vi "G#Object_Create.vi"(0 "reference in":refnum<class "G#BaseAggregator.lvclass">, 3 "control values":variant[](array[variant]), 5 "error in (no error)":errorcluster) -> (14 "reference out":refnum<class "G#BaseAggregator.lvclass">, 19 "error out":errorcluster)   [LabVIEW 2017, in "G#BaseAggregator.lvclass"]
uses:
  G#BaseAggregator.lvclass
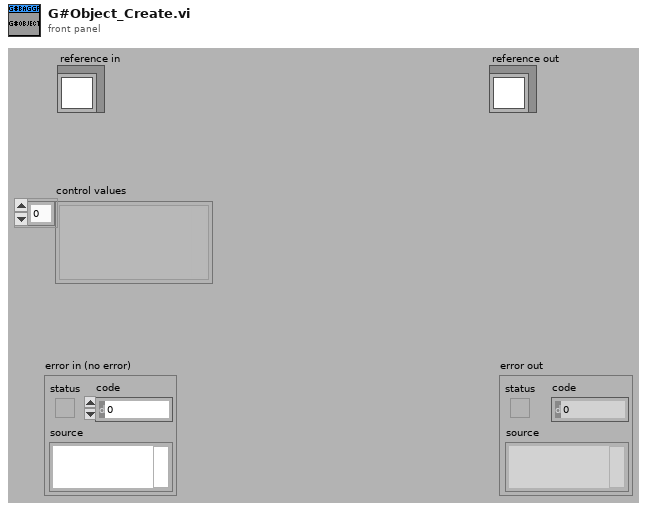
[diagram p1: front panel]
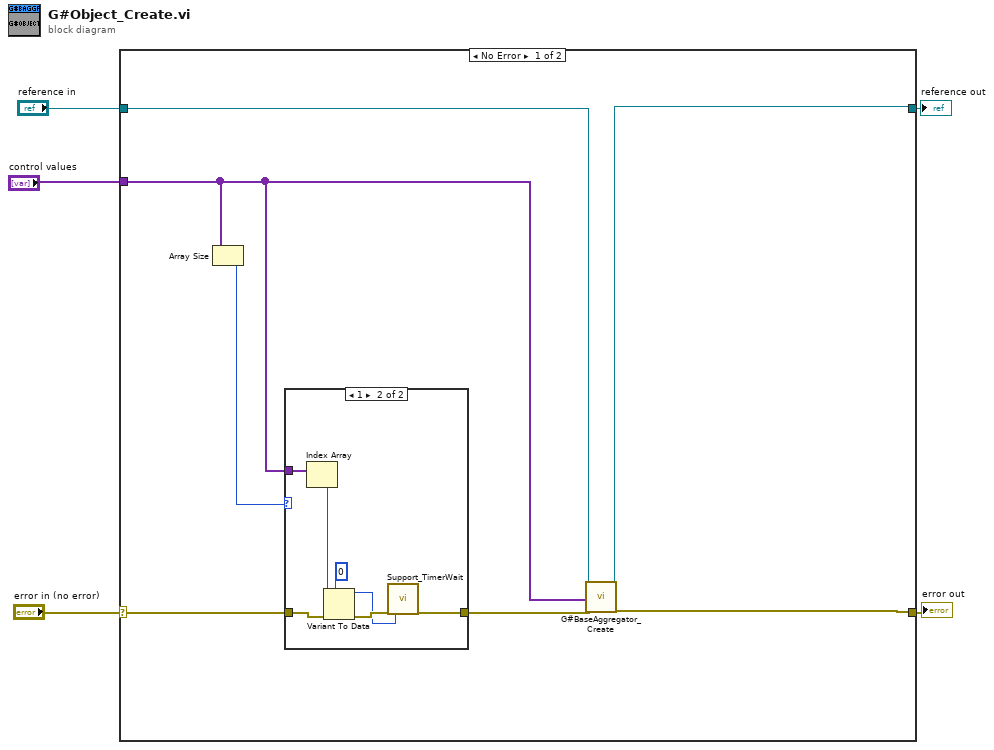
[diagram p0: block diagram]
diagram:
  n1 = case shown="No Error" "error in (no error)" {
    selector: "error in (no error)" -> [w8 w22]
    tunnel: [w10 w22] -> w4
    tunnel: [w11 w21] -> w2
    tunnel: "reference in" -> [w12 w21]
    tunnel: "control values" -> [w6 _]
    frame No Error {
      n2 = Array Size(array=w6) -> (size(s)=w9:i32)
      n3 = case shown="1" w9 {
        tunnel: w8 -> [w13 w20]
        tunnel: [w13 w17] -> w7
        tunnel: w6 -> [_ w18]
        frame 0, Default {
        }
        frame 1 {
          n4 = Index Array(array=w18) -> (element=w19:variant)  [unwired: 1 in]
          n5 = Variant To Data(error in=w20, type=u32 0 ("milliseconds to wait"), Variant=w19) -> (data=w14:u32, error out=w16:errorcluster)
          n6 = call "Support_TimerWait.vi"("error in (no error)"=w16, "milliseconds to wait"=w14) -> ("error out"=w17:errorcluster)  [unwired: 17 in]
        }
      }
      n7 = call "G#BaseAggregator_Create.vi"("reference in"=w12, "control values"=w6, "error in (no error)"=w7) -> ("reference out"=w11:refnum<class "G#BaseAggregator.lvclass">, "error out"=w10:errorcluster)  [unwired: 15 in]
    }
    frame Error {
    }
  }
  "error out" <- w4
  "reference out" <- w2
